vi "Intake & Transfer Controller.vi"(8 "error in":errorcluster) -> ()   [LabVIEW 2019]
doc: "This VI executes continuously carrying out the current operation and responding to updates or new operations. It will often contain the timing or control code that is difficult to place directly in TeleOp. This VI generally opens all sensors and motors and isolates the rest of the robot code from knowing how the operations are carried out."
uses:
  <vilib>/Rock Robotics/WPI/Framework/Completion Status.ctl
  Intake & Transfer Setpoints.ctl
  Intake & Transfer Operations.ctl
  <vilib>/Rock Robotics/SystemInterfaces/DIO/FPGA_DIOChannel.ctl
  <vilib>/Rock Robotics/WPI/ThirdParty/REV Robotics/SPARK MAX/Typedef/Spark MAX Idle Mode.ctl
  <vilib>/Rock Robotics/WPI/ThirdParty/REV Robotics/SPARK MAX/Typedef/Spark MAX Control Type.ctl
  <vilib>/Rock Robotics/WPI/Switch/WPI_SwitchOpenLimit.vi
  Framework/Robot Global Data.vi
  <vilib>/Rock Robotics/Network Tables/NT Write Boolean.vi
panel:
  out "Waveform Chart":dbl(graph)
  in  "Transfer Reset":dbl=-0.25
  in  "Transfer Forward Slow":dbl=0.1
  in  "Transfer Rev slow":dbl=-0.15
  in  "Transfer Rev Fast":dbl=-0.15
  in  "Intake Timer":u32
  in  "Wait time":u32=200
  in  "Reset Max Delay":u32=1000
  in  "Reset Min Delay":u32=500
  in  "Transfer Forward Power":dbl=0.2
  in  "Interactive Values":T1
  out "Current\nCmd":string
  in  "Buttons":cluster{"Execute Cmd":bool, "Abort Cmd":bool}
  out "Command Timing":cluster{"Start Time (ms)":u32, "Iterations":i32}
  out "Status":T3
  # "Tip: It may be helpful to observe inputs and sensor values.\nYou may also want to display tuning or debugging controls."
  # "Reset"
  # "0 .. 2"
  # "State 3"
  # "Interactive Command: You may fill in the settings for a command\nand schedule it with the Execute button. You can observe and abort\nany command while fine tuning the code for the controller."
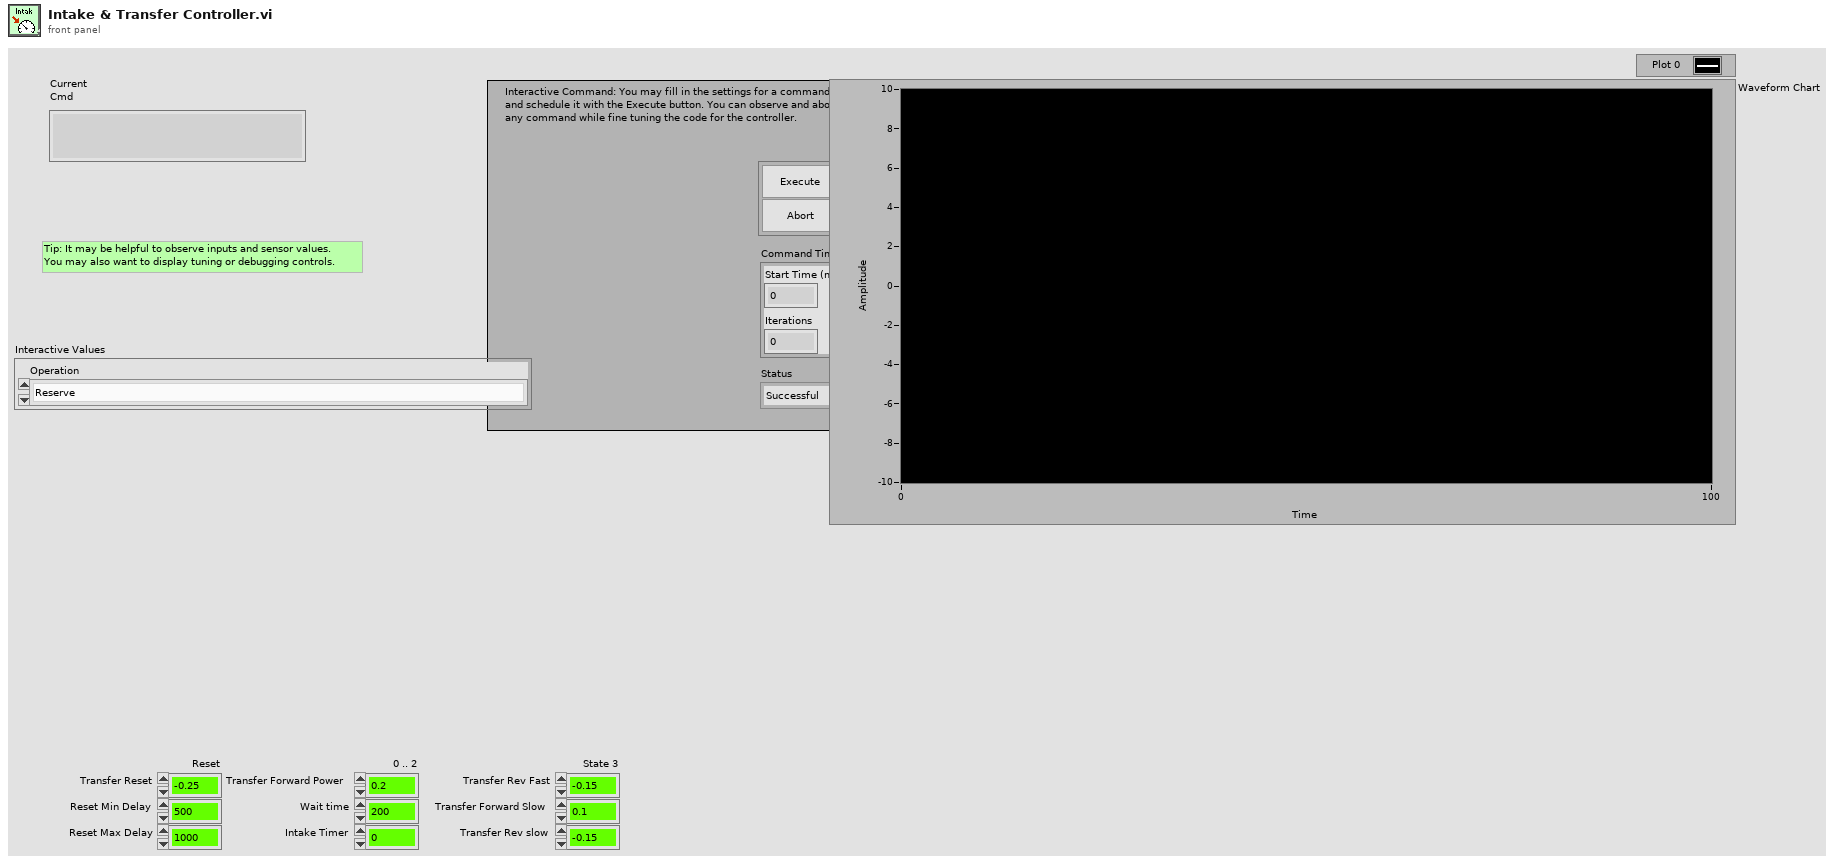
[diagram p1: front panel]
types:
  T1 = typedef "Intake & Transfer Setpoints.ctl" = cluster{"Operation":T2}
  T2 = typedef "Intake & Transfer Operations.ctl" = enum16{"Reserve", "Read Current", "Ready"}
  T3 = typedef "Completion Status.ctl" = enum16{"Successful", "Aborted", "Incomplete"}
  T4 = cluster{"P Gain":dbl, "I Gain":dbl, "D Gain":dbl, "F Gain":dbl, "I Zone":dbl, "Min Output":dbl, "Max Output":dbl}
  T5 = typedef "Spark MAX Idle Mode.ctl" = enum16{"Coast", "Brake"}
  T6 = typedef "FPGA_DIOChannel.ctl" = enum8{"DIO 0", "DIO 1", "DIO 2", "DIO 3", "DIO 4", "DIO 5", "DIO 6", "DIO 7", "DIO 8", "DIO 9", "DIO MXP 0", "DIO MXP 1", "DIO MXP 2", "DIO MXP 3", "DIO MXP 4", "DIO MXP 5", "DIO MXP 6", "DIO MXP 7", "DIO MXP 8", "DIO MXP 9", "DIO MXP 10", "DIO MXP 11", "DIO MXP 12", "DIO MXP 13", "DIO MXP 14", "DIO MXP 15", "SPI Port CS1", "SPI Port CS2", "SPI Port CS3", "SPI Port MISO", "SPI Port MOSI", "Invalid"}
  T7 = typedef "WPI_MotorControlDeviceRef.ctl" = cluster{"DeviceStatus":errorcluster, "Type":T8, "PWM":cluster{"PWM Channel":T9, "DeadBand":T10}, "CAN":cluster{"Device Number":u8, "SetOutput VI Ref":variant, "GetOutput VI Ref":variant, "Enable VI Ref":variant, "Disable VI Ref":variant, "Data":variant}, "Invert":bool, "DIO PWM":cluster{"PWM \"Enable\" Channel":T9, "DIOChannel":T6, "PWM Rate":dbl}}
  T8 = typedef "WPI_MotorControlType.ctl" = enum16{"PWM", "CAN", "DIO PWM"}
  T9 = typedef "FPGA_DIOPWMChannel.ctl" = enum8{"PWM 0", "PWM 1", "PWM 2", "PWM 3", "PWM 4", "PWM 5", "PWM 6", "PWM 7", "PWM 8", "PWM 9", "PWM MXP 0", "PWM MXP 1", "PWM MXP 2", "PWM MXP 3", "PWM MXP 4", "PWM MXP 5", "PWM MXP 6", "PWM MXP 7", "PWM MXP 8", "PWM MXP 9", "Invalid"}
  T10 = typedef "WPI_PWMDeadband.ctl" = cluster{"Name":string, "maxPositivePwm":i32, "minPositivePwm":i32, "centerPwm":i32, "maxNegativePwm":i32, "minNegativePwm":i32, "angularRange":u16}
  T11 = typedef "WPI_SwitchDevRef.ctl" = cluster{"DevStatus":errorcluster, "DIO Channel":T6, "CntIndex":T12, "Normally Closed":bool}
  T12 = typedef "FPGA_CounterCtrSystemIndex.ctl" = enum8{"Ctr 0", "Ctr 1", "Ctr 2", "Ctr 3", "Ctr 4", "Ctr 5", "Ctr 6", "Ctr 7", "Invalid"}
  T13 = typedef "Command Status Info.ctl" = cluster{"Name":string, "Status":T3, "notifier out":T14}
  T14 = typedef "Completion Notifier.ctl" = refnum<notifier>
  T15 = cluster{"Current Command":T1, "Command Timing":cluster{"Start Time (ms)":u32, "Iterations":i32}, "Command Arguments":cluster{"Command Info":T13, "Description":string, "Default Command":T1, "queue out":refnum<queue>, "Subsystem Name":string}}
  T16 = typedef "Spark MAX Control Type.ctl" = enum16{"Percent VBus", "Voltage", "Velocity", "Position", "Smart Motion", "Current", "Smart Velocity"}
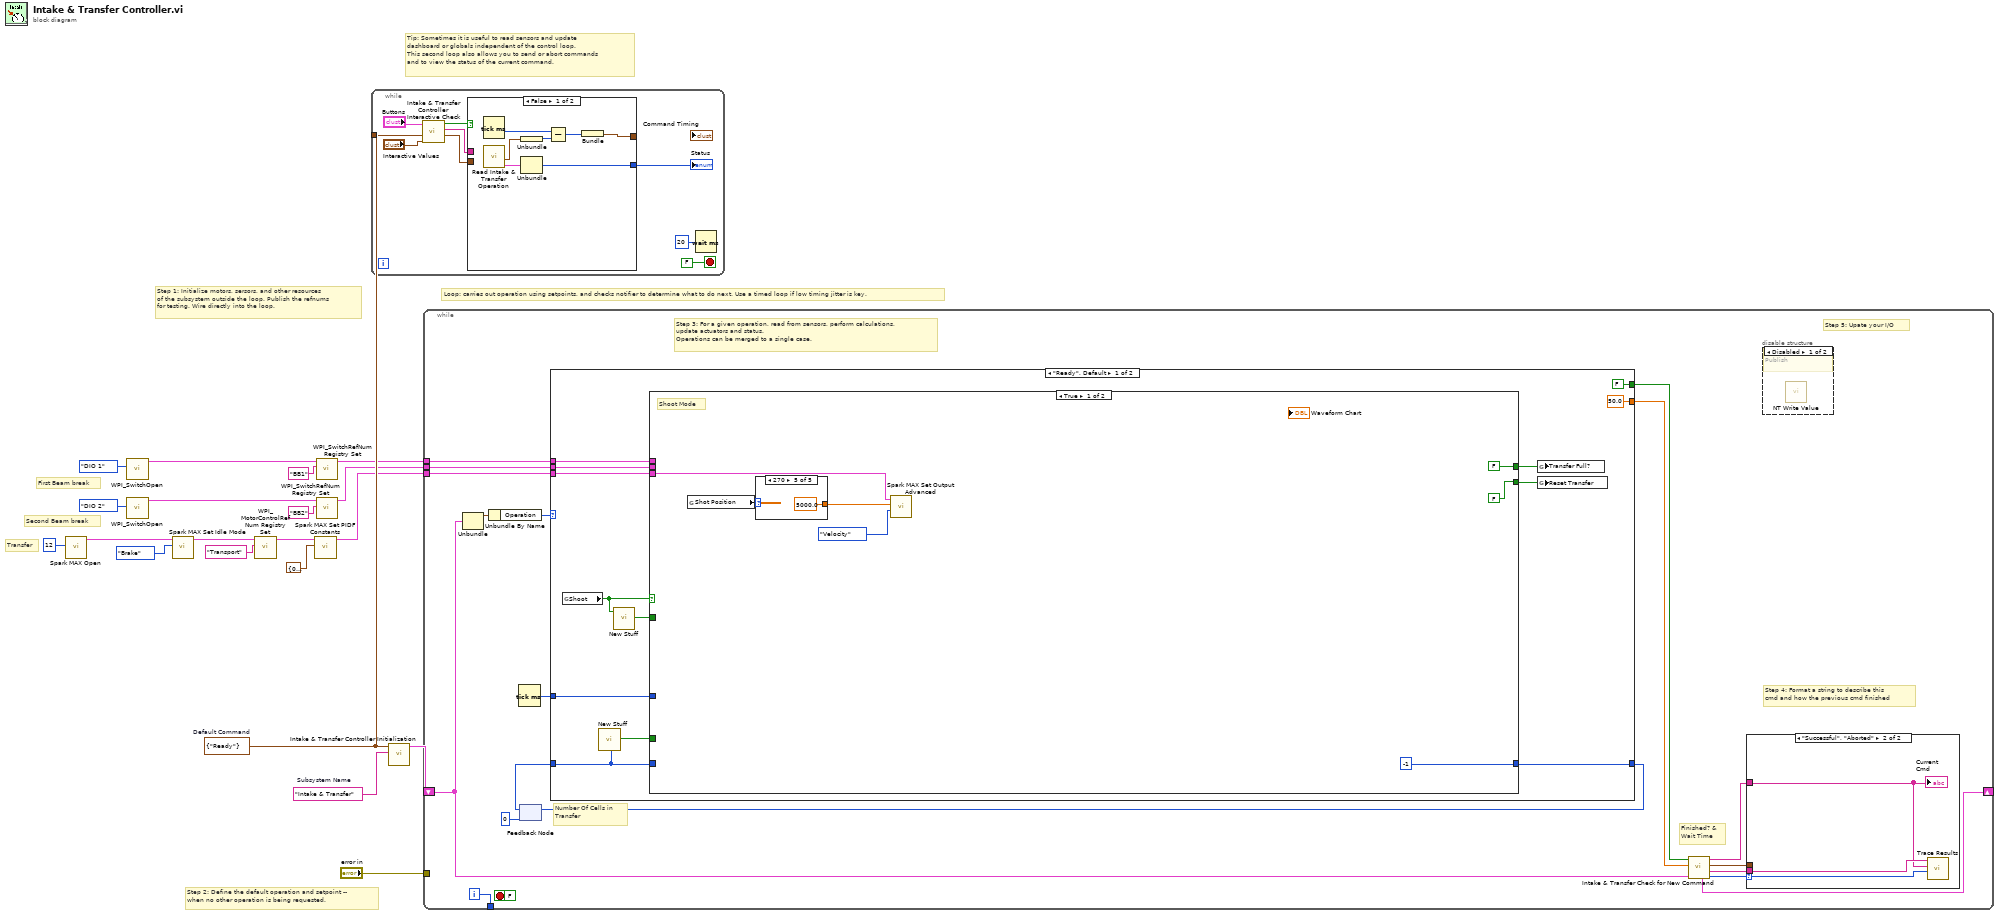
[diagram p0: block diagram]
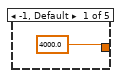
[diagram p2: hidden frame]
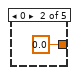
[diagram p3: hidden frame]
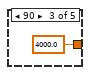
[diagram p4: hidden frame]
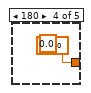
[diagram p5: hidden frame]
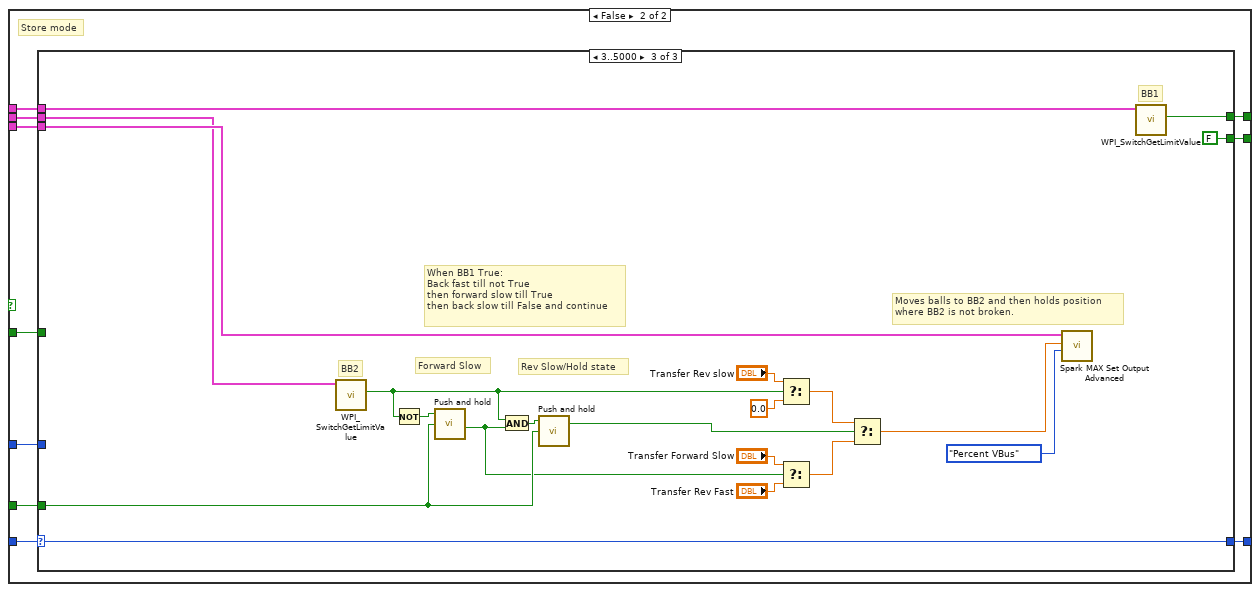
[diagram p6: hidden frame]
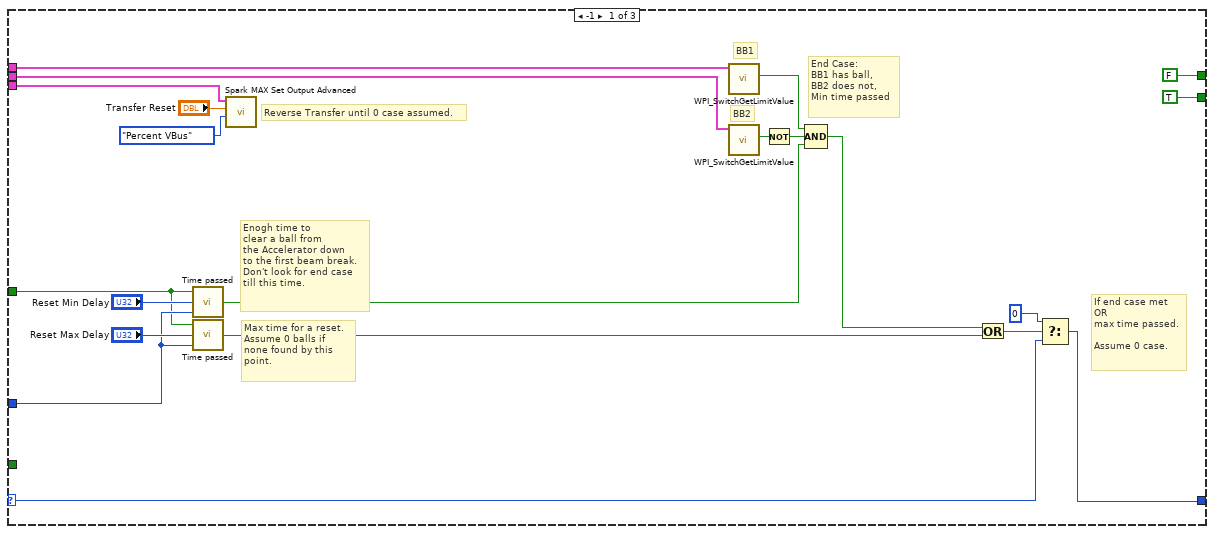
[diagram p7: hidden frame]
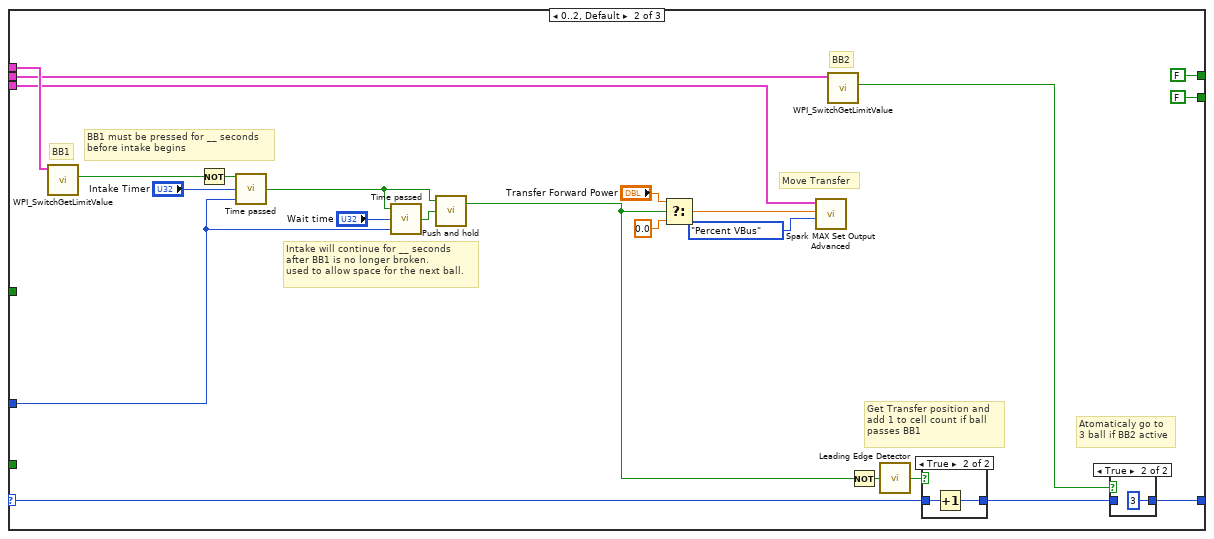
[diagram p8: hidden frame]
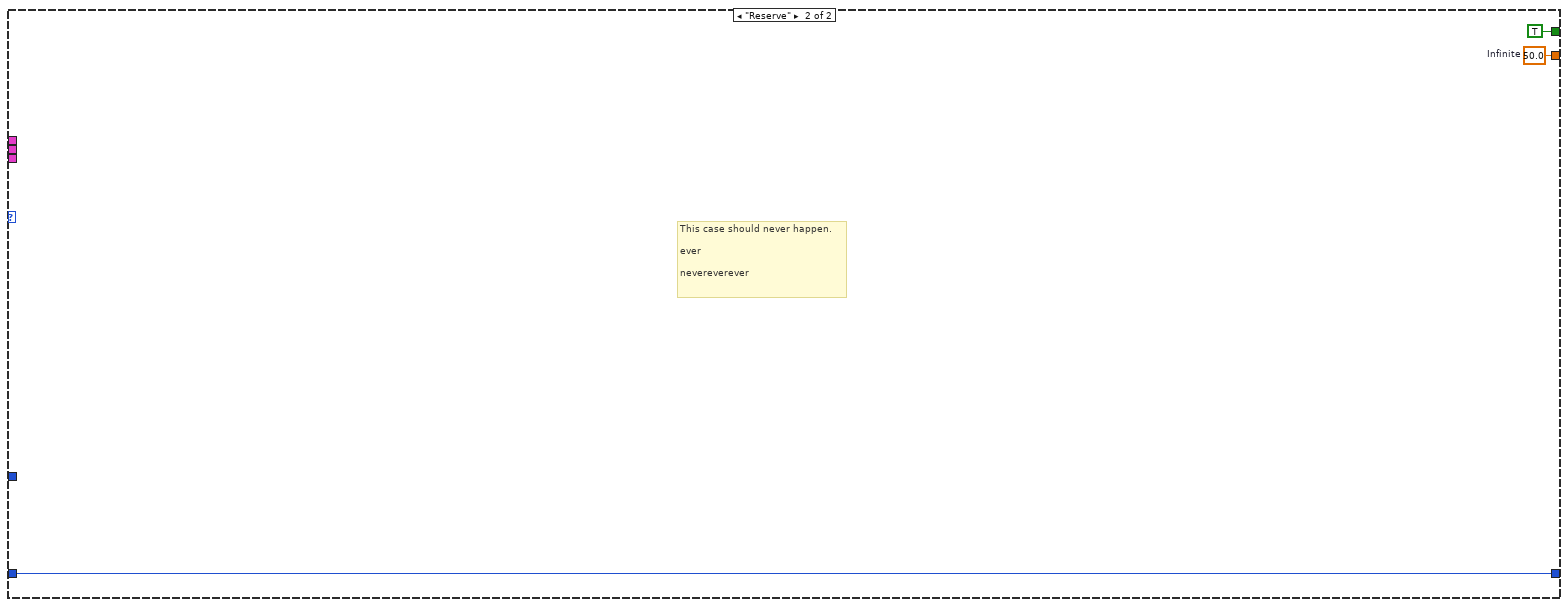
[diagram p11: hidden frame]
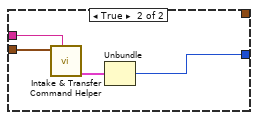
[diagram p14: hidden frame]
diagram:
  w17 = T1 {"Operation"=enum."Ready"}  # Default Command
  w18 = "Intake & Transfer"  # Subsystem Name
  # "Second Beam break"
  # "First Beam break"
  # "Transfer"
  # "Tip: Sometimes it is useful to read sensors and update\ndashboard or globals independent of the control loop.\nThis second loop also allows you to send or abort commands\nand to view the status of the current command."
  # "Step 2: Define the default operation and setpoint --\nwhen no other operation is being requested."
  # "Step 1: Initialize motors, sersors, and other resources\nof the subsystem outside the loop. Publish the refnums\nfor testing. Wire directly into the loop."
  # "Loop: carries out operation using setpoints, and checks notifier to determine what to do next. Use a timed loop if low timing jitter is key."
  n1 = call <vilib>:"Spark MAX Open.vi"("Device Number"=u8 12) -> ("MotorControlDeviceRef"=w6:T7)  [unwired: 9 in, 1 out]
  n2 = call-poly <vilib>:"WPI_SwitchOpen.vi"("DIO Channel"=FPGA_DIOChannel."DIO 1") -> ("SwitchDevRef"=w15:T11)  [unwired: 9 in, 1 out]
  n3 = call-poly <vilib>:"WPI_SwitchOpen.vi"("DIO Channel"=FPGA_DIOChannel."DIO 2") -> ("SwitchDevRef"=w7:T11)  [unwired: 9 in, 1 out]
  n4 = call <vilib>:"Spark MAX Set Idle Mode.vi"("Idle Mode"=Spark_MAX_Idle_Mode."Brake", "MotorControlDeviceRef in"=w6) -> ("MotorControlDeviceRef out"=w4:T7)  [unwired: 8 in, 1 out]
  n5 = call <vilib>:"WPI_MotorControlRefNum Registry Set.vi"("refnum name"="Transport", "MotorControlDevRef"=w4) -> ("MotorControlDevRef"=w3:T7)  [unwired: 8 in, 1 out]
  n6 = call <vilib>:"Spark MAX Set PIDF Constants.vi"("PID Constants"=T4 {"P Gain"=0.0001, "I Gain"=0.0, "D Gain"=0.0, "F Gain"=0.00015, "I Zone"=0.0, "Min Output"=-1.0, "Max Output"=1.0}, "MotorControlDeviceRef"=w3) -> ("MotorControlDeviceRef"=w2:T7)  [unwired: 8 in, 1 out]
  n7 = call <vilib>:"WPI_SwitchRefNum Registry Set.vi"("refnum name"="BB1", "SwitchDevRef"=w15) -> ("SwitchDevRef"=w12:T11)  [unwired: 8 in, 1 out]
  n8 = call <vilib>:"WPI_SwitchRefNum Registry Set.vi"("refnum name"="BB2", "SwitchDevRef"=w7) -> ("SwitchDevRef"=w11:T11)  [unwired: 8 in, 1 out]
  n9 = while {
    tunnel: w17 -> [w26]
    stop <- FALSE stop-if-true
    n10 = call "Intake & Transfer Controller Interactive Check.vi"("Interactive Command in"="Interactive Values", "Default Command"=w26, "Buttons"="Buttons") -> ("Interactive Command out"=w23:T1, "Trace String"=w24:string, "Schedule"=w25:bool)  [unwired: 6 in]
    n11 = case shown="False" w25 {
      tunnel: [w36 w40] -> w22
      tunnel: w23 -> [_ w38]
      tunnel: [w33 _] -> _
      tunnel: w24 -> [_ w39]
      frame False {
        n12 = Tick Count (ms)() -> (millisecond timer value=w32:u32)
        n13 = call "Read Intake & Transfer Operation.vi"() -> ("Command Info"=w30:T13, "SubSystem Data"=w31:T1)  [unwired: 9 in, 1 out]
        n14 = Unbundle(w31) -> ("Operation"=w35:T2)
        n15 = Unbundle(w30) -> ("Status"=w36:T3)  [unwired: 2 out]
        n16 = Subtract(x=w32, y=w35) -> (x-y=w34:u32)
        n17 = Bundle(w34) -> (w33:cluster{u32})  [unwired: 1 in]
      }
      frame True {
        n18 = call "Intake & Transfer Command Helper.vi"("Description"=w39, "SubSystem Data"=w38) -> ("Command Info Out"=w37:T13)  [unwired: 7 in, 2 out]
        n19 = Unbundle(w37) -> ("Status"=w40:T3)  [unwired: 2 out]
      }
    }
    "Status" <- w22
    n20 = Wait (ms)(milliseconds to wait=u32 20) -> ()  [unwired: 1 out]
  }
  n21 = call "Intake & Transfer Controller Initialization.vi"("Subsystem Name"=w18, "Default Command"=w17) -> ("Current Command"=w19:T15)  [unwired: 9 in]
  n22 = while {
    shift-right: [w54] -> _
    shift-left: w19 -> [w47]
    tunnel: [w58] -> _
    tunnel: "error in" -> [_]
    tunnel: w12 -> [w43]
    tunnel: w11 -> [w42]
    tunnel: w2 -> [w41]
    i -> [w58]
    stop <- FALSE stop-if-true
    # "Number Of Cells in\nTransfer"
    # "Step 5: Upate your I/O"
    # "Step 4: Format a string to describe this\ncmd and how the previous cmd finished"
    # "Finished? &\nWait Time"
    # "Step 3: For a given operation, read from sensors, perform calculations,\nupdate actuators and status.\nOperations can be merged to a single case."
    n23 = Unbundle(w47) -> ("Current Command"=w57:T1)  [unwired: 2 out]
    n24 = Unbundle By Name(w57) -> ("Operation"=w56:T2)
    n25 = Tick Count (ms)() -> (millisecond timer value=w55:u32)
    n26 = feedback #1(i64 0) -> (w45:i64)
    n27 = case shown="\"Ready\", Default" w56 {
      tunnel: [50.0 ("Infinite") w166] -> w52
      tunnel: [FALSE ("ignore previous (F)") TRUE ("ignore previous (F)")] -> w53
      tunnel: w55 -> [w69 _]
      tunnel: [w70 w164] -> w46
      tunnel: w45 -> [w61 w164]
      tunnel: w43 -> [w72 _]
      tunnel: w42 -> [w71 _]
      tunnel: w41 -> [w66 _]
      frame "Ready", Default {
        n28 = global read "Robot Global Data.vi" "Shoot"() -> (w64:bool)
        n29 = call "New Stuff.vi"("Variant 9"=w61) -> ("x != y?"=w60:bool)  [unwired: 26 in]
        n30 = call "New Stuff.vi"("Variant 2"=w64) -> ("x != y?"=w65:bool)  [unwired: 26 in]
        n31 = case shown="True" w64 {
          tunnel: w72 -> [_ w94]
          tunnel: w71 -> [_ w93]
          tunnel: w66 -> [w75 w92]
          tunnel: [i64 -1 ("t") w91] -> w70
          tunnel: w69 -> [_ w90]
          tunnel: w61 -> [_ w89]
          tunnel: w65 -> [_ w86]
          tunnel: [FALSE ("Switch Pressed") w88] -> w63
          tunnel: [FALSE ("Switch Pressed") w87] -> w62
          tunnel: w60 -> [_ w85]
          frame True {
            # "Shoot Mode"
            n32 = global read "Robot Global Data.vi" "Shot Position"() -> (w74:dbl)
            n33 = case shown="270" w74 {
              tunnel: [4000.0 ("Numeric") 0.0 ("Numeric") 4000.0 ("Numeric") 0.0 ("Numeric") 5000.0] -> w73
              frame -1, Default {
              }
              frame 0 {
              }
              frame 90 {
              }
              frame 180 {
                (unwired) 4000.0 ("Numeric")
              }
              frame 270 {
              }
            }
            n34 = call <vilib>:"Spark MAX Set Output Advanced.vi"("Control Mode"=Spark_MAX_Control_Type."Velocity", "Setpoint"=w73, "MotorControlDevRef"=w75) -> ()  [unwired: 7 in, 2 out]
          }
          frame False {
            # "Store mode"
            n35 = case shown="3..5000" w89 {
              selector: w89 -> [w110 w138 w161]
              tunnel: w94 -> [w114 w137 w160]
              tunnel: w93 -> [w115 w116 w162]
              tunnel: w92 -> [w103 w119 w163]
              tunnel: [w99 w136 w161] -> w91
              tunnel: w90 -> [w104 w127 _]
              tunnel: [FALSE ("Switch Pressed") FALSE ("Switch Pressed") w159] -> w88
              tunnel: [TRUE ("Switch Pressed") FALSE ("Switch Pressed") FALSE ("Switch Pressed")] -> w87
              tunnel: w86 -> [w96 _ _]
              tunnel: w85 -> [_ _ w155]
              frame -1 {
                # "Reverse Transfer until 0 case assumed."
                # "End Case:\nBB1 has ball,\nBB2 does not,\nMin time passed"
                # "If end case met \nOR\nmax time passed.\n\nAssume 0 case."
                # "BB2"
                # "BB1"
                # "Max time for a reset. \nAssume 0 balls if \nnone found by this \npoint."
                # "Enogh time to \nclear a ball from \nthe Accelerator down \nto the first beam break. \nDon't look for end case \ntill this time."
                n36 = call "Time passed.vi"("ms timer value"=w104, "Wait time"="Reset Min Delay", "Reset"=w96) -> ("Boolean out"=w106:bool)
                n37 = call "Time passed.vi"("ms timer value"=w104, "Wait time"="Reset Max Delay", "Reset"=w96) -> ("Boolean out"=w102:bool)
                n38 = call <vilib>:"Spark MAX Set Output Advanced.vi"("Control Mode"=Spark_MAX_Control_Type."Percent VBus", "Setpoint"="Transfer Reset", "MotorControlDevRef"=w103) -> ()  [unwired: 7 in, 2 out]
                n39 = call <vilib>:"WPI_SwitchGetLimitValue.vi"("SwitchDevRef"=w114) -> ("Switch Pressed"=w112:bool)  [unwired: 8 in, 2 out]
                n40 = call <vilib>:"WPI_SwitchGetLimitValue.vi"("SwitchDevRef"=w115) -> ("Switch Pressed"=w113:bool)  [unwired: 8 in, 2 out]
                n41 = Not(x=w113) -> (.not. x?=w111:bool)
                n42 = Compound Arithmetic op=AND(w112, w111, w106) -> (w101:bool)
                n43 = Or(x=w101, y=w102) -> (x .or. y?=w100:bool)
                n44 = Select(t=i64 0, s=w100, f=w110) -> (s? t:f=w99:i64)
              }
              frame 0..2, Default {
                # "Intake will continue for __ seconds\nafter BB1 is no longer broken.\nused to allow space for the next ball."
                # "BB1 must be pressed for __ seconds\nbefore intake begins"
                # "Atomaticaly go to\n3 ball if BB2 active"
                # "BB2"
                # "BB1"
                # "Get Transfer position and \nadd 1 to cell count if ball \npasses BB1"
                # "Move Transfer"
                n45 = call <vilib>:"WPI_SwitchGetLimitValue.vi"("SwitchDevRef"=w137) -> ("Switch Pressed"=w128:bool)  [unwired: 8 in, 2 out]
                n46 = Not(x=w128) -> (.not. x?=w129:bool)
                n47 = call "Time passed.vi"("ms timer value"=w127, "Wait time"="Intake Timer", "Reset"=w129) -> ("Boolean out"=w125:bool)
                n48 = call "Time passed.vi"("ms timer value"=w127, "Wait time"="Wait time", "Reset"=w125) -> ("Boolean out"=w130:bool)
                n49 = call "Push and hold.vi"("Reset"=w130, "Input"=w125) -> ("Output"=w118:bool)  [unwired: 2 in]
                n50 = Select(t="Transfer Forward Power", s=w118, f=0.0 ("Setpoint")) -> (s? t:f=w117:dbl)
                n51 = call <vilib>:"Spark MAX Set Output Advanced.vi"("Control Mode"=Spark_MAX_Control_Type."Percent VBus", "Setpoint"=w117, "MotorControlDevRef"=w119) -> ()  [unwired: 7 in, 2 out]
                n52 = call <vilib>:"WPI_SwitchGetLimitValue.vi"("SwitchDevRef"=w116) -> ("Switch Pressed"=w134:bool)  [unwired: 8 in, 2 out]
                n53 = Not(x=w118) -> (.not. x?=w133:bool)
                n54 = call "Leading Edge Detector.vi"("Boolean"=w133) -> ("Out"=w132:bool)
                n55 = case shown="True" w132 {
                  tunnel: w138 -> [w141 w143]
                  tunnel: [w141 w142] -> w135
                  frame False {
                  }
                  frame True {
                    n56 = Increment(x=w143) -> (x+1=w142:i64)
                  }
                }
                n57 = case shown="True" w134 {
                  tunnel: [w139 i64 3] -> w136
                  tunnel: w135 -> [w139 _]
                  frame False {
                  }
                  frame True {
                  }
                }
              }
              frame 3..5000 {
                # "When BB1 True:\nBack fast till not True\nthen forward slow till True\nthen back slow till False and continue"
                # "BB2"
                # "Rev Slow/Hold state"
                # "Forward Slow"
                # "BB1"
                # "Moves balls to BB2 and then holds position\nwhere BB2 is not broken."
                n58 = call <vilib>:"WPI_SwitchGetLimitValue.vi"("SwitchDevRef"=w162) -> ("Switch Pressed"=w148:bool)  [unwired: 8 in, 2 out]
                n59 = Not(x=w148) -> (.not. x?=w157:bool)
                n60 = call "Push and hold.vi"("Reset"=w155, "Input"=w157) -> ("Output"=w152:bool)  [unwired: 2 in]
                n61 = And(x=w148, y=w152) -> (x .and. y?=w156:bool)
                n62 = call "Push and hold.vi"("Reset"=w155, "Input"=w156) -> ("Output"=w150:bool)  [unwired: 2 in]
                n63 = Select(t="Transfer Rev slow", s=w148, f=0.0 ("Setpoint")) -> (s? t:f=w145:dbl)
                n64 = Select(t="Transfer Forward Slow", s=w152, f="Transfer Rev Fast") -> (s? t:f=w149:dbl)
                n65 = Select(t=w145, s=w150, f=w149) -> (s? t:f=w144:dbl)
                n66 = call <vilib>:"Spark MAX Set Output Advanced.vi"("Control Mode"=Spark_MAX_Control_Type."Percent VBus", "Setpoint"=w144, "MotorControlDevRef"=w163) -> ()  [unwired: 7 in, 2 out]
                n67 = call <vilib>:"WPI_SwitchGetLimitValue.vi"("SwitchDevRef"=w160) -> ("Switch Pressed"=w159:bool)  [unwired: 8 in, 2 out]
              }
            }
          }
        }
        n68 = global write "Robot Global Data.vi" "Transfer Full?"(w63) -> ()
        n69 = global write "Robot Global Data.vi" "Reset Transfer"(w62) -> ()
      }
      frame "Reserve" {
        w166 = 50.0  # Infinite
        # "This case should never happen.\n\never\n\nnevereverever"
      }
    }
    n70 = feedback-in #1(w46) -> ()
    n71 = call "Intake & Transfer Check for New Command.vi"("Current Command"=w47, "Wait time (ms)"=w52, "Finished?"=w53) -> ("Completion"=w48:T3, "Subsystem Name"=w49:string, "Current Command"=w50:T1, "Initial Trace String"=w51:string, "NextCommand"=w54:T15)  [unwired: 4 in]
    n72 = case shown="\"Successful\", \"Aborted\"" w48 {
      selector: w48 -> [_ w169]
      tunnel: w51 -> [_ w167]
      tunnel: w50 -> [_ _]
      tunnel: w49 -> [_ w168]
      frame "Incomplete", Default {
        # "Continuing current command"
      }
      frame "Successful", "Aborted" {
        # "Report and setup for next command"
        n73 = call <vilib>:"Trace Results.vi"("Status of previous command"=w169, "Description"=w167, "Subsystem"=w168) -> ()  [unwired: 9 in]
        "Current\nCmd" <- w167
      }
    }
    n74 = disable-structure shown="Disabled" {
      frame Disabled {
        # "Publish"
        n75 = call-poly <vilib>:"NT Write Value.vi"() -> ()  [unwired: 11 in, 1 out]
      }
      frame Enabled {
      }
    }
  }
